vi "Overlap Adjustment.vi"(8 "Error In":errorcluster, 11 "Overlap (%)":dbl) -> (0 "Error Out":errorcluster, 3 "Overlap Adjustment (0-1)":dbl)   [LabVIEW 2014]
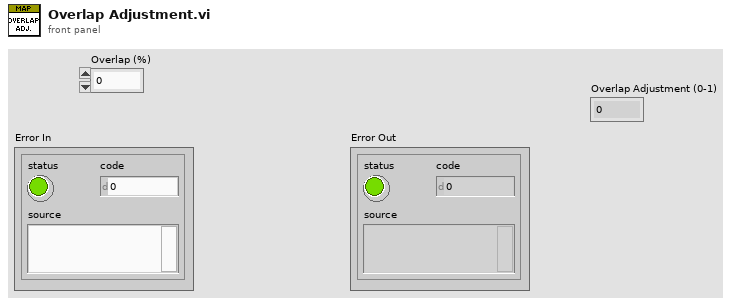
[diagram p1: front panel]
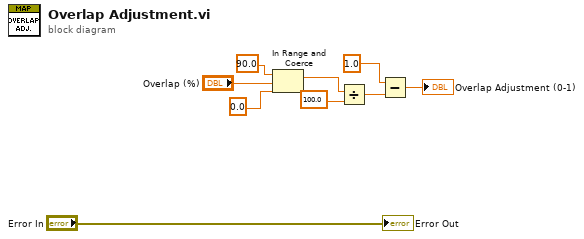
[diagram p0: block diagram]
diagram:
  n1 = In Range and Coerce(upper limit=90.0, x="Overlap (%)", lower limit=0.0) -> (coerced(x)=w6:dbl)  [unwired: 1 out]
  n2 = Divide(x=w6, y=100.0) -> (x/y=w9:dbl)
  n3 = Subtract(x=1.0, y=w9) -> (x-y=→"Overlap Adjustment (0-1)":dbl)
  "Error Out" <- "Error In"
